vi "Time String(ms).vi"() -> (2 "system time string(ms)":string)   [LabVIEW 2020]
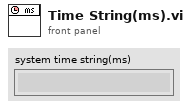
[diagram p1: front panel]
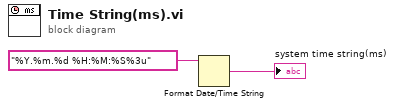
[diagram p0: block diagram]
diagram:
  n1 = Format Date/Time String(time format string (%c)="%Y.%m.%d %H:%M:%S%3u") -> (date/time string=→"system time string(ms)":string)  [unwired: 2 in]
